vi "ReadFile.vi"(11 "String":string) -> (2 "file contents":string, 3 "reply":string)   [LabVIEW 2019]
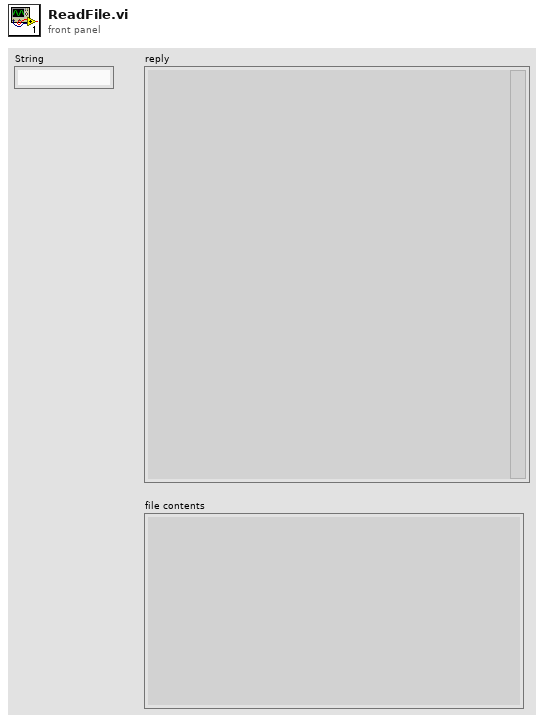
[diagram p1: front panel]
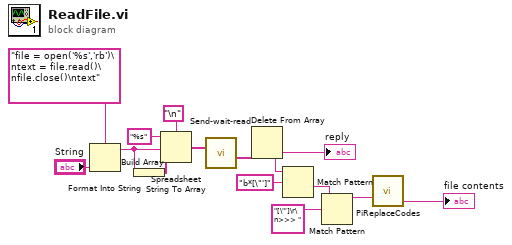
[diagram p0: block diagram]
diagram:
  n1 = Format Into String(format string="file = open('%s','rb')\ntext = file.read()\nfile.close()\ntext" ("write buffer"), "String") -> (resulting string=w3:string)  [unwired: 2 in, 1 out]
  n2 = Build Array(w3) -> (w4:string[])
  n3 = Spreadsheet String To Array(delimiter (Tab)="\n", format string="%s", spreadsheet string=w3, array type (2D Dbl)=w4) -> (array=w7:string[])
  n4 = call "Send-wait-read.vi"("commands"=w7) -> ("All strings"=w11:string[])  [unwired: 9 in, 1 out]
  n5 = Delete From Array(array=w11) -> (deleted portion=w12:string)  [unwired: 2 in, 1 out]
  "reply" <- w12
  n6 = Match Pattern(string=w12, regular expression="b*[\"']") -> (after substring=w9:string)  [unwired: 1 in, 3 out]
  n7 = Match Pattern(string=w9, regular expression="[\"']\r\n>>> ") -> (before substring=w13:string)  [unwired: 1 in, 3 out]
  n8 = call "PiReplaceCodes.vi"("Conv String in"=w13) -> ("String out"=→"file contents":string)  [unwired: 9 in, 1 out]
